vi "getEvents.vi"(8 "error in (no error)":errorcluster, 11 "CameraEventsManger in":refnum<class "CameraEventsManger.lvclass">) -> (0 "error out":errorcluster, 1 "cameraSettingsEventsRef":T3, 2 "settingsEvents":T1, 3 "CameraEventsManger out":refnum<class "CameraEventsManger.lvclass">, 4 "snapperEvents":T2)   [LabVIEW 2009, in "Tools.lvlib" / "Settings.lvlib" / "CameraEventsManger.lvclass"]
uses:
  CameraEventsManger.lvclass
  CameraSettingsEventsManager/cameraSettingsEventManager.lvclass
  CameraEventsManger.lvclass/CameraEventsManger.ctl
  Viewers/Snapper/SnapperEvents.lvclass
  Tools/SettingsEventManager/SettingsEventsManager.lvclass
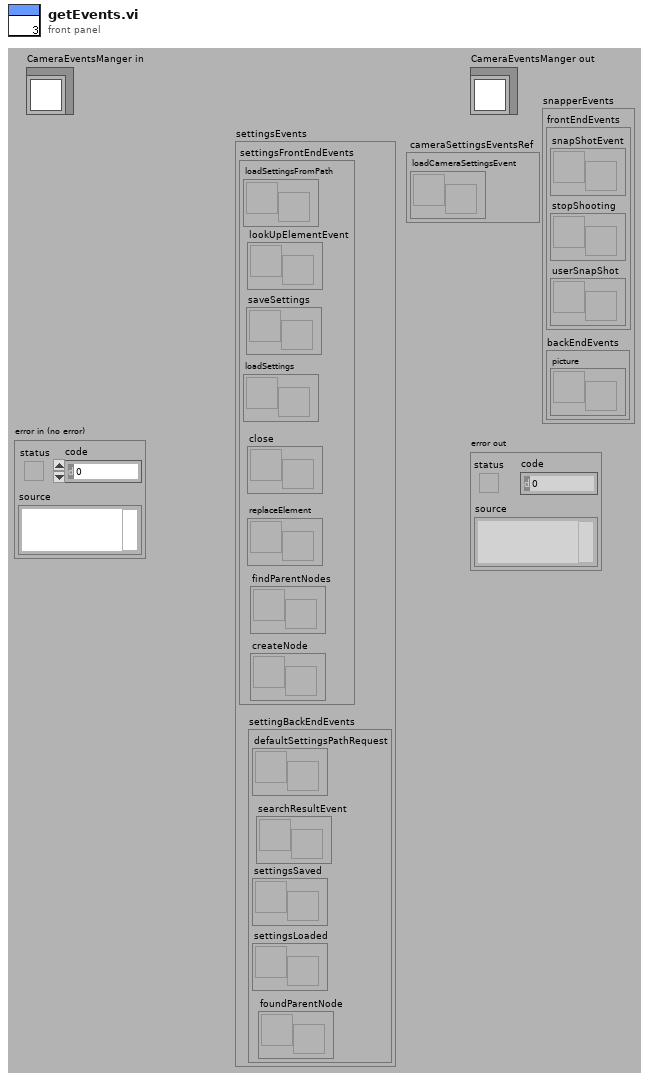
[diagram p1: front panel]
types:
  T1 = cluster{"settingsFrontEndEvents":cluster{"loadSettingsFromPath":refnum<user-event>, "lookUpElementEvent":refnum<user-event>, "saveSettings":refnum<user-event>, "loadSettings":refnum<user-event>, "close":refnum<user-event>, "replaceElement":refnum<user-event>, "findParentNodes":refnum<user-event>, "createNode":refnum<user-event>}, "settingBackEndEvents":cluster{"defaultSettingsPathRequest":refnum<user-event>, "searchResultEvent":refnum<user-event>, "settingsSaved":refnum<user-event>, "settingsLoaded":refnum<user-event>, "foundParentNode":refnum<user-event>}}
  T2 = cluster{"frontEndEvents":cluster{"snapShotEvent":refnum<user-event>, "stopShooting":refnum<user-event>, "userSnapShot":refnum<user-event>}, "backEndEvents":cluster{"picture":refnum<user-event>}}
  T3 = cluster{"loadCameraSettingsEvent":refnum<user-event>}
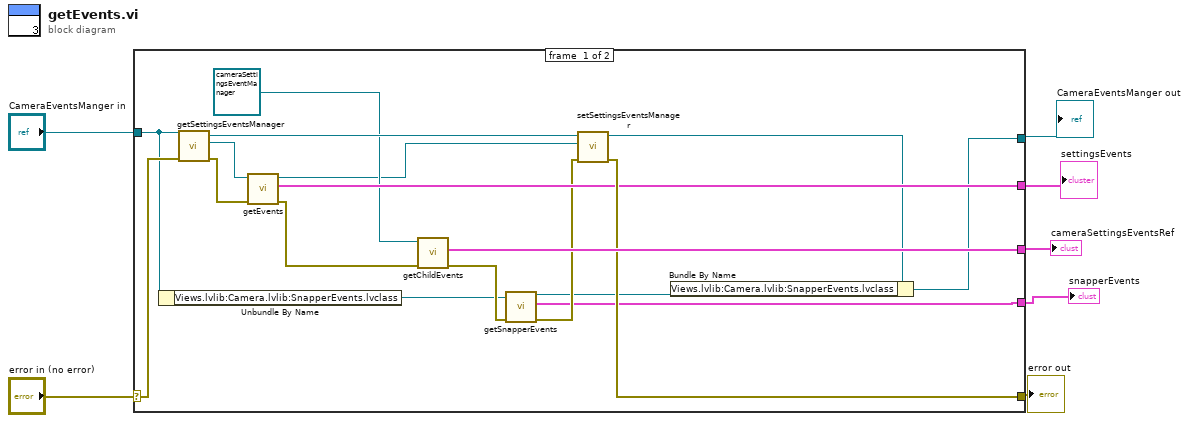
[diagram p0: block diagram]
diagram:
  n1 = case shown="No Error" "error in (no error)" {
    selector: "error in (no error)" -> [w25 w27]
    tunnel: [w20 w27] -> w6
    tunnel: [w12 w26] -> w4
    tunnel: "CameraEventsManger in" -> [w17 w26]
    tunnel: [w19 _] -> w1
    tunnel: [w22 _] -> w3
    tunnel: [w11 _] -> w2
    frame #0 {
      n2 = Unbundle By Name(w17) -> ("Views.lvlib:Camera.lvlib:SnapperEvents.lvclass"=w16:refnum<class "SnapperEvents.lvclass">)
      n3 = call-dynamic "getSettingsEventsManager.vi"("error in (no error)"=w25, "CameraEventsManger.lvclass in"=w17) -> ("error out"=w23:errorcluster, "SettingsEventsManager"=w24:refnum<class "SettingsEventsManager.lvclass">, "CameraEventsManger.lvclass out"=w21:refnum<class "CameraEventsManger.lvclass">)  [unwired: 7 in]
      n4 = call-dynamic "getEvents.vi"("error in (no error)"=w23, "SettingsEventsManager in"=w24) -> ("error out"=w10:errorcluster, "settingsEvents"=w19:T1, "SettingsEventsManager out"=w8:refnum<class "SettingsEventsManager.lvclass">)  [unwired: 7 in]
      n5 = call-dynamic "getChildEvents.vi"("error in (no error)"=w10, "cameraSettingsEventManager in"=refnum<class "cameraSettingsEventManager.lvclass"> refnum ("Hardware:Channels.lvlib:cameraSettingsEventManager.lvclass")) -> ("error out"=w18:errorcluster, "cameraSettingsEventsRef"=w22:T3)  [unwired: 7 in, 1 out]
      n6 = call-dynamic "getSnapperEvents.vi"("error in (no error)"=w18, "SnapperEvents in"=w16) -> ("error out"=w15:errorcluster, "snapperEvents"=w11:T2, "SnapperEvents out"=w14:refnum<class "SnapperEvents.lvclass">)  [unwired: 7 in]
      n7 = call-dynamic "setSettingsEventsManager.vi"("error in (no error)"=w15, "Tools.lvlib:Settings.lvlib:SettingsEventsManager.lvclass"=w8, "CameraEventsManger.lvclass in"=w21) -> ("error out"=w20:errorcluster, "CameraEventsManger.lvclass out"=w13:refnum<class "CameraEventsManger.lvclass">)  [unwired: 7 in]
      n8 = Bundle By Name(cluster=w13, "Views.lvlib:Camera.lvlib:SnapperEvents.lvclass"=w14) -> (w12:refnum<class "CameraEventsManger.lvclass">)
    }
    frame #1 {
    }
  }
  "error out" <- w6
  "CameraEventsManger out" <- w4
  "cameraSettingsEventsRef" <- w3
  "snapperEvents" <- w2
  "settingsEvents" <- w1
